vi "calc_polarization.vi"(1 "Time (seconds)":i64, 2 "Rate (k)":dbl, 3 "Exp coefficient (C)":dbl, 4 "Steady state (A)":dbl) -> (0 "Polarization (raw)":dbl)   [LabVIEW 2010]
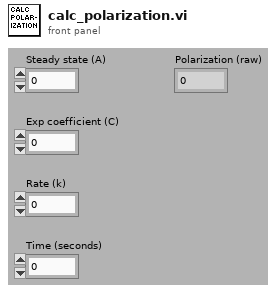
[diagram p1: front panel]
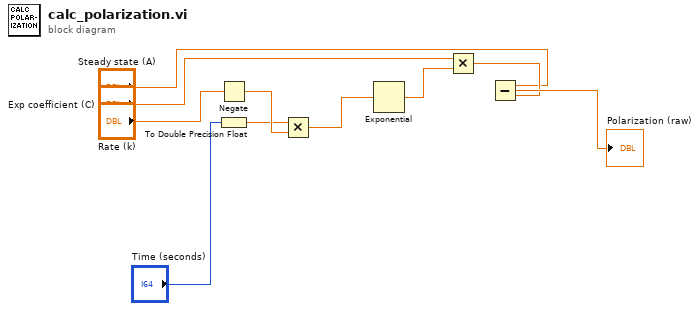
[diagram p0: block diagram]
diagram:
  n1 = Negate(x="Rate (k)") -> (-x=w9:dbl)
  n2 = To Double Precision Float(number="Time (seconds)") -> (double precision float=w6:dbl)
  n3 = Multiply(x=w6, y=w9) -> (x*y=w7:dbl)
  n4 = Exponential(1:w7) -> (0:w4:dbl)
  n5 = Multiply(x="Exp coefficient (C)", y=w4) -> (x*y=w3:dbl)
  n6 = Subtract(x="Steady state (A)", y=w3) -> (x-y=→"Polarization (raw)":dbl)
